vi "Configure Trigger at Beginning of Step.vi"(8 "error in (no error)":errorcluster, 10 "Trigger Outputs At Beginning Of Steps":bool[](array[boolean]), 11 "VISA resource name":refnum<visa-resource-name>) -> (0 "error out":errorcluster, 3 "VISA resource name out":refnum<visa-resource-name>)   [LabVIEW 2019, in "Agilent N7976A.lvlib"]
doc: "Specifies which list steps generate a trigger signal at the beginning of step. The trigger signal can be used as a trigger source for measurements and transients of other units, and for digital port pins configured as trigger outputs."
uses:
  <instrlib>/Agilent N7976A/Agilent N7976A.lvlib
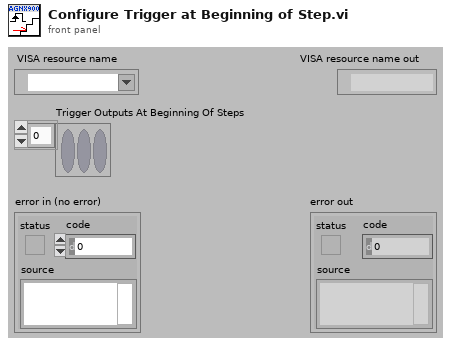
[diagram p1: front panel]
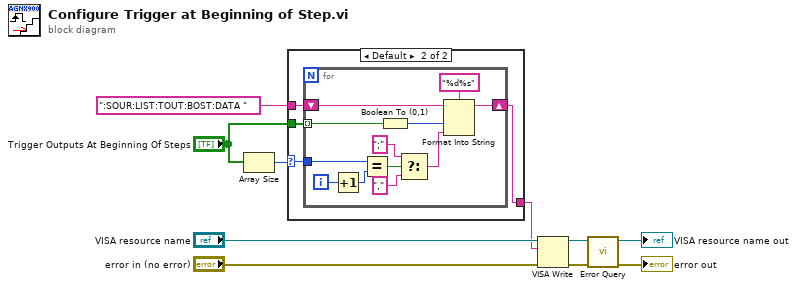
[diagram p0: block diagram]
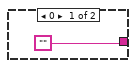
[diagram p2: hidden frame]
diagram:
  n1 = Array Size(array="Trigger Outputs At Beginning Of Steps") -> (size(s)=w4:i32)
  n2 = case shown="Default" w4 {
    selector: w4 -> [_ w13]
    tunnel: "Trigger Outputs At Beginning Of Steps" -> [_ w14]
    tunnel: ":SOUR:LIST:TOUT:BOST:DATA " -> [_ w15]
    tunnel: ["" w12] -> w1
    frame 0 {
    }
    frame Default {
      n3 = for {
        shift-right: [w16] -> w12
        shift-left: w15 -> [w21]
        tunnel: w14 -> [w18] mode=indexing
        tunnel: w13 -> [w25]
        i -> [w27]
        n4 = Increment(x=w27) -> (x+1=w26:i32)
        n5 = Equal?(x=w25, y=w26) -> (x = y?=w24:bool)
        n6 = Boolean To (0,1)(Boolean=w18) -> (0, 1=w19:i16)
        n7 = Select(t=";", s=w24, f=",") -> (s? t:f=w20:string)
        n8 = Format Into String(format string="%d%s", initial string=w21, w19, w20) -> (resulting string=w16:string)  [unwired: 1 in, 1 out]
      }
    }
  }
  n9 = VISA Write(VISA resource name="VISA resource name", write buffer=w1, error in (no error)="error in (no error)") -> (VISA resource name out=w7:refnum<visa-resource-name>, error out=w8:errorcluster)  [unwired: 1 out]
  n10 = call <instrlib>:"Error Query.vi"("error in (no error)"=w8, "VISA resource name"=w7) -> ("error out"=→"error out":errorcluster, "VISA resource name out"=→"VISA resource name out":refnum<visa-resource-name>)  [unwired: 6 in, 2 out]
